vi "stand_alone_host.vi"() -> ()   [LabVIEW 2021]
uses:
  <vilib>/userdefined/High Color/nirio_resource_hc.ctl
  outside/pulse_gen_and_detect_p2p/pulse_gen_and_detect_p2p.lvclass
panel:
  out "amp / f":cluster{"X":dbl, "Y":dbl}[](graph)
  out "PW/f":cluster{"X":dbl, "Y":dbl}[](graph)
  out "PW":dbl[](graph)
  out "AMP":dbl[](graph)
  out "size(s)":i32
  out "t / f":cluster{"X":dbl, "Y":dbl}[](graph)
  in  "num of pulses to read":i64=-1
  out "error out":errorcluster={"status"=TRUE, "code"=-63192, "source"="niLvFpga_Open_PXIe-5785 (KU060).vi:2790006"}
  in  "user configurations":T2={"vst_device"=["VST_1", "VST_2"], "RF gain "=10.0, "buffer size"=524288, "center frequency (Hz) "=1000000000.0, "P2P sample rate"=200000000.0, "mode"=enum."5785 - 2*180MHz", "devicess"=["IF_transceiver_2"], "file paths"=[path "C:/Users/PXIe8108_Demo/Documents/CHAIM DATA/chaim/5785_sync_for_elbit/data/pdw_test_file.tdms", path "C:/Users/PXIe8108_Demo/Documents/CHAIM DATA/chaim/5785_sync_for_elbit/data/pdw_test_file_1.tdms", path "C:/Users/PXIe8108_Demo/Documents/CHAIM DATA/chaim/5785_sync_for_elbit/data/pdw_test_file_2.tdms", path "C:/Users/PXIe8108_Demo/Documents/CHAIM DATA/chaim/5785_sync_for_elbit/data/pdw_test_file_3.tdms", path "C:/Users/PXIe8108_Demo/Documents/CHAIM DATA/chaim/5785_sync_for_elbit/data/pdw_test_file_4.tdms"], "gen for df"=FALSE} {"buffer size" step=512}
  in  "stop":bool
  out "Current DDS Allocation":bool[][](array[boolean])
  out "Pulse transmited":u32(slide) max=1210602 scale=0.0..13783.0 scale format="%#_3p"
  out "Elapsed Time (sec)":dbl format="%#.1g"
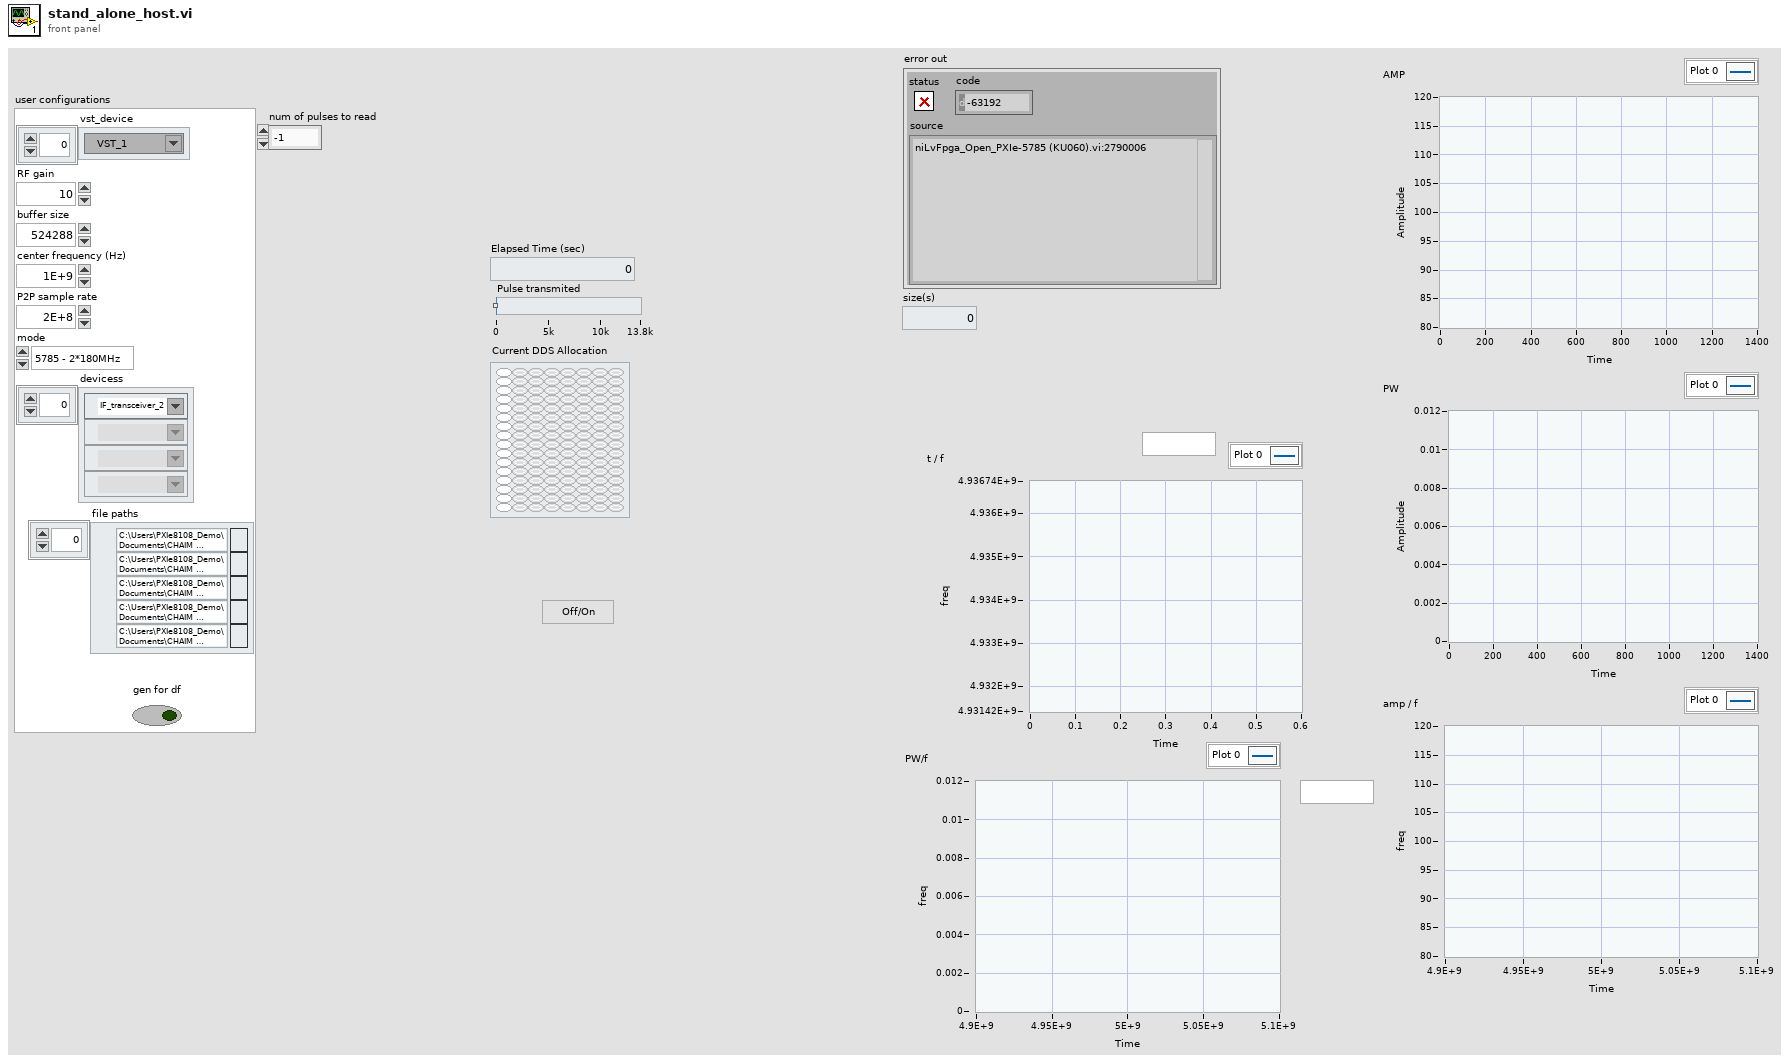
[diagram p1: front panel]
types:
  T1 = typedef "nirio_resource_hc.ctl" = tag
  T2 = cluster{"vst_device":refnum<k15>[], "RF gain ":dbl, "buffer size":u32, "center frequency (Hz) ":dbl, "P2P sample rate":dbl, "mode":enum16{"USRP - 180MHz", "5785 - 2*180MHz", "5785 - 3.2GHz", "P2P - VST"}, "devicess":T1[], "file paths":path[], "gen for df":bool}
  T3 = cluster{"fpga clock":dbl, "pulse transmitted":u32, "dds free":bool[][]}
  T4 = cluster{"f":dbl, "pw":dbl, "amp":dbl, "tend":dbl}[]
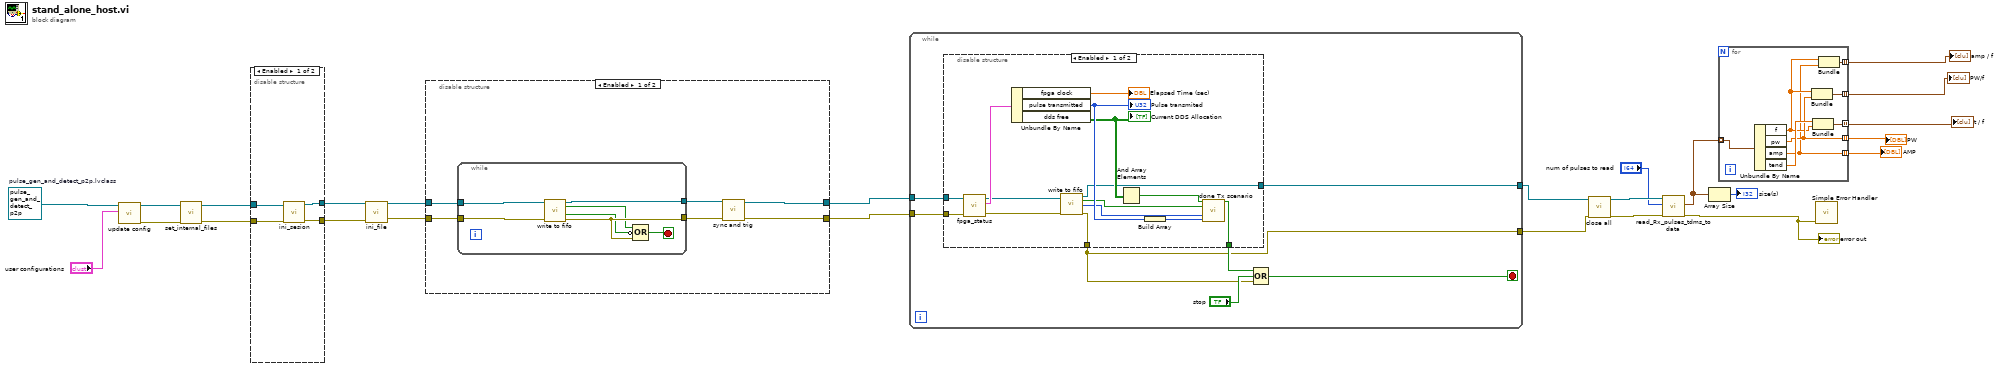
[diagram p0: block diagram]
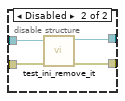
[diagram p3: hidden frame]
diagram:
  w25 = refnum<class "pulse_gen_and_detect_p2p.lvclass"> refnum  # pulse_gen_and_detect_p2p.lvclass
  n1 = call-dynamic "update config.vi"("user configurations"="user configurations", "pulse_gen_and_detect_p2p in"=w25) -> ("error out"=w23:errorcluster, "pulse_gen_and_detect_p2p out"=w24:refnum<class "pulse_gen_and_detect_p2p.lvclass">)  [unwired: 6 in, 2 out]
  n2 = call-dynamic "set_internal_files.vi"("error in (no error)"=w23, "pulse_gen_and_detect_p2p in"=w24) -> ("error out"=w19:errorcluster, "pulse_gen_and_detect_p2p out"=w20:refnum<class "pulse_gen_and_detect_p2p.lvclass">)  [unwired: 8 in]
  n3 = disable-structure shown="Enabled" {
    disable-tunnel: [w29 w30] -> w22
    disable-tunnel: [w28 w31] -> w21
    disable-tunnel: w20 -> [w27 w33]
    disable-tunnel: w19 -> [w26 w32]
    frame Enabled {
      n4 = call-dynamic "ini_sesion.vi"("error in (no error)"=w26, "pulse_gen_and_detect_p2p in"=w27) -> ("error out"=w28:errorcluster, "pulse_gen_and_detect_p2p out"=w29:refnum<class "pulse_gen_and_detect_p2p.lvclass">)  [unwired: 8 in]
    }
    frame Disabled {
      n5 = call "test_ini_remove_it.vi"("error in"=w32, "pulse_gen_and_detect_p2p out"=w33) -> ("error out"=w31:errorcluster, "pulse_gen_and_detect_p2p out 2"=w30:refnum<class "pulse_gen_and_detect_p2p.lvclass">)  [unwired: 8 in]
    }
  }
  n6 = call-dynamic "ini_file.vi"("device_type in"=w22, "error in (no error)"=w21) -> ("device_type out"=w18:refnum<class "pulse_gen_and_detect_p2p.lvclass">, "error out"=w17:errorcluster)  [unwired: 11 in, 1 out]
  n7 = disable-structure shown="Enabled" {
    disable-tunnel: w18 -> [w39 w48]
    disable-tunnel: w17 -> [w38 w47]
    disable-tunnel: [w35 w48] -> w16
    disable-tunnel: [w34 w47] -> w15
    frame Enabled {
      n8 = while {
        tunnel: w39 -> [w46]
        tunnel: w38 -> [w45]
        tunnel: [w44] -> w37
        tunnel: [w42] -> w36
        stop <- w43 stop-if-true
        n9 = call-dynamic "write to fifo.vi"("pulse_gen_and_detect_p2p in"=w46, "error in (no error)"=w45) -> ("pulse_gen_and_detect_p2p out"=w44:refnum<class "pulse_gen_and_detect_p2p.lvclass">, "done write file"=w40:bool, "room on fifo"=w41:bool, "error out"=w42:errorcluster)  [unwired: 9 in, 1 out]
        n10 = Compound Arithmetic op=OR(w40, invert w41, w42) -> (w43:bool)
      }
      n11 = call-dynamic "sync and trig.vi"("error in (no error)"=w36, "pulse_gen_and_detect_p2p in"=w37) -> ("error out"=w34:errorcluster, "pulse_gen_and_detect_p2p out"=w35:refnum<class "pulse_gen_and_detect_p2p.lvclass">)  [unwired: 8 in]
    }
    frame Disabled {
    }
  }
  n12 = while {
    tunnel: w16 -> [w55]
    tunnel: w15 -> [w54]
    tunnel: [w50] -> w14
    tunnel: [w49] -> w13
    stop <- w53 stop-if-true
    n13 = disable-structure shown="Enabled" {
      disable-tunnel: w55 -> [w60 w71]
      disable-tunnel: w54 -> [w59 _]
      disable-tunnel: [w58 _] -> w52
      disable-tunnel: [w57 w71] -> w50
      disable-tunnel: [w56 _] -> w49
      frame Enabled {
        n14 = call-dynamic "fpga_status.vi"("error in (no error)"=w59, "pulse_gen_and_detect_p2p in"=w60) -> ("error out"=w67:errorcluster, "pulse TX status"=w70:T3, "pulse_gen_and_detect_p2p out"=w68:refnum<class "pulse_gen_and_detect_p2p.lvclass">)  [unwired: 7 in]
        n15 = Unbundle By Name(w70) -> ("fpga clock"=→"Elapsed Time (sec)":dbl, "pulse transmitted"=w66:u32, "dds free"=w62:bool[][])
        "Pulse transmited" <- w66
        "Current DDS Allocation" <- w62
        n16 = call-dynamic "write to fifo.vi"("pulse_gen_and_detect_p2p in"=w68, "error in (no error)"=w67) -> ("pulse_gen_and_detect_p2p out"=w57:refnum<class "pulse_gen_and_detect_p2p.lvclass">, "done write file"=w63:bool, "num of pulses sent to the FPGA"=w64:u32, "error out"=w56:errorcluster)  [unwired: 9 in, 1 out]
        n17 = And Array Elements(Boolean array=w62) -> (logical AND=w61:bool)
        n18 = Build Array(w66) -> (w65:u32[])
        n19 = call "done Tx scenario.vi"("all dds free"=w61, "done write files"=w63, "num of pulse sent to fpga"=w64, "pulse transmitted"=w65) -> ("Done Tx secenario?"=w58:bool)  [unwired: 11 in]
      }
      frame Disabled {
      }
    }
    n20 = Compound Arithmetic op=OR(w52, "stop", w49) -> (w53:bool)
  }
  n21 = call-dynamic "close all.vi"("error in (no error)"=w13, "pulse_gen_and_detect_p2p in"=w14) -> ("error out"=w11:errorcluster, "pulse_gen_and_detect_p2p out"=w9:refnum<class "pulse_gen_and_detect_p2p.lvclass">)  [unwired: 8 in]
  n22 = call-dynamic "read_Rx_pulses_tdms_to data.vi"("error in (no error)"=w11, "num of pulses to read"="num of pulses to read", "pulse_gen_and_detect_p2p in"=w9) -> ("error out"=w10:errorcluster, "PDWout"=w6:T4)  [unwired: 6 in, 1 out]
  "error out" <- w10
  n23 = Array Size(array=w6) -> (size(s)=→"size(s)":i32)
  n24 = for {
    tunnel: w6 -> [w79] mode=indexing
    tunnel: [w78] -> w7 mode=indexing
    tunnel: [w73] -> w4 mode=indexing
    tunnel: [w76] -> w3 mode=indexing
    tunnel: [w75] -> w2 mode=indexing
    tunnel: [w72] -> w1 mode=indexing
    n25 = Unbundle By Name(w79) -> ("f"=w74:dbl, "pw"=w76:dbl, "amp"=w73:dbl, "tend"=w77:dbl)
    n26 = Bundle("f"=w74, "pw"=w76) -> (w75:cluster{"f":dbl, "pw":dbl})  [unwired: 1 in]
    n27 = Bundle("tend"=w77, "f"=w74) -> (w78:cluster{"tend":dbl, "f":dbl})  [unwired: 1 in]
    n28 = Bundle("f"=w74, "amp"=w73) -> (w72:cluster{"f":dbl, "amp":dbl})  [unwired: 1 in]
  }
  "t / f" <- w7
  "AMP" <- w4
  "PW" <- w3
  "PW/f" <- w2
  "amp / f" <- w1
  n29 = call <vilib>:"Simple Error Handler.vi"("error in (no error)"=w10) -> ()  [unwired: 4 in, 5 out]
